vi "FPGA - Clear.vi"(8 "error in (no error)":errorcluster, 11 "Node Ptr":u64 format="%.0x") -> (0 "error out":errorcluster)   [LabVIEW 2011, in "Scan Engine Custom Device.lvlib"]
uses:
  Scan Engine Custom Device.lvlib
  Type Defs/FPGA Target.ctl
  Type Defs/Host - FPGAScanInterfaceMode.ctl
  Globals/Scan Engine GUIDs.vi
  <vilib>/NI Veristand/Custom Device API/Custom Device API.lvlib
  <vilib>/NI Veristand/Custom Device Tools/Custom Device Utility Library/Custom Device Utility Library.lvlib
panel:
  in  "Tag":string
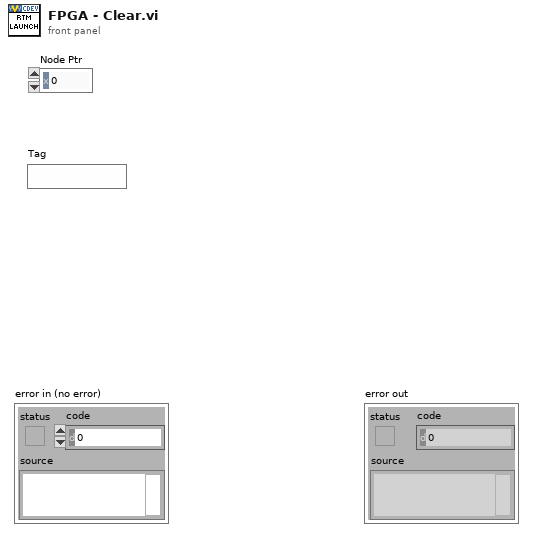
[diagram p1: front panel]
types:
  T1 = typedef "Scan Engine Custom Device.lvlib/Host - FPGAScanInterfaceMode.ctl" = enum16{"Use Current", "FPGA", "Scan Mode"}
  T2 = typedef "Scan Engine Custom Device.lvlib/FPGA Target.ctl" = enum16{"Local", "EtherCAT"}
  T3 = typedef "Custom Device API.lvlib/Custom Device Item Info.ctl" = cluster{"Name":string, "Is Channel":bool, "GUID":string}
  T4 = typedef "Custom Device API.lvlib/Custom Device Item Ref.ctl" = u64
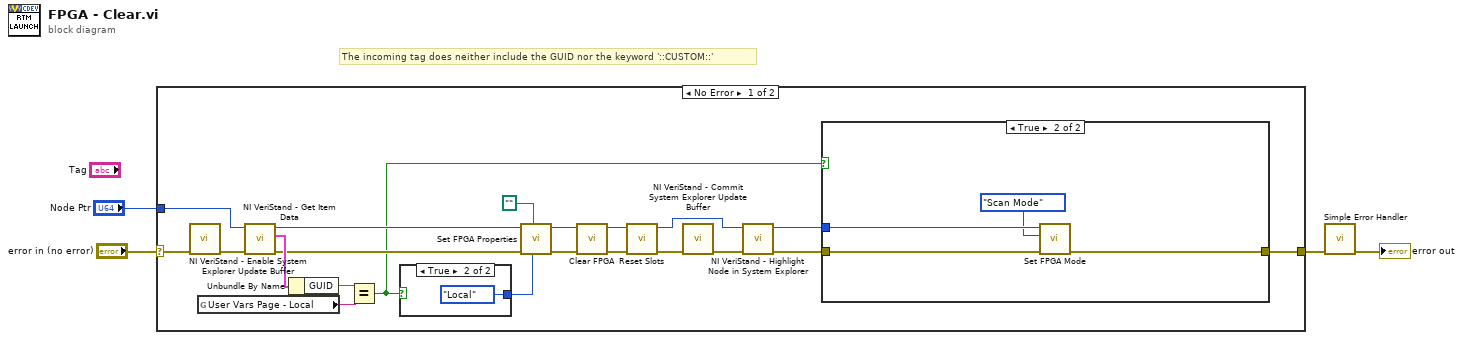
[diagram p0: block diagram]
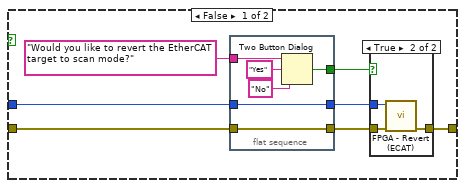
[diagram p2: hidden frame]
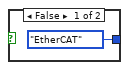
[diagram p4: hidden frame]
diagram:
  # "The incoming tag does neither include the GUID nor the keyword '::CUSTOM::'"
  n1 = case shown="No Error" "error in (no error)" {
    selector: "error in (no error)" -> [w19 w49]
    tunnel: "Node Ptr" -> [w13 _]
    tunnel: [w6 w49] -> w2
    frame No Error {
      n2 = call <vilib>:"NI VeriStand - Enable System Explorer Update Buffer.vi"("error in (no error)"=w19) -> ("error out"=w14:errorcluster)  [unwired: 10 in]
      n3 = global read "Scan Engine GUIDs.vi" "User Vars Page - Local"() -> (w10:string)
      n4 = call <vilib>:"NI VeriStand - Get Item Data.vi"("error in (no error)"=w14, "Item Ref in"=w13) -> ("error out"=w9:errorcluster, "Item Info"=w15:T3, "Item Ref out"=w12:T4)  [unwired: 6 in, 1 out]
      n5 = Unbundle By Name(w15) -> ("GUID"=w11:string)
      n6 = Equal?(x=w11, y=w10) -> (x = y?=w5:bool)
      n7 = case shown="True" w5 {
        tunnel: [FPGA_Target."EtherCAT" ("FPGA Target") FPGA_Target."Local" ("FPGA Target")] -> w23
        frame False {
        }
        frame True {
        }
      }
      n8 = call "Set FPGA Properties.vi"("FPGA Target"=w23, "Bitfile Path"=path "", "error in (no error)"=w9, "Item Ref in"=w12) -> ("error out"=w20:errorcluster, "Item Ref out"=w21:T4)  [unwired: 6 in]
      n9 = call "Clear FPGA.vi"("error in (no error)"=w20, "Item Ref in"=w21) -> ("error out"=w24:errorcluster, "Item Ref out"=w25:T4)  [unwired: 8 in]
      n10 = call "Reset Slots.vi"("error in (no error)"=w24, "Item Ref in"=w25) -> ("error out"=w18:errorcluster, "Item Ref out"=w16:T4)  [unwired: 8 in]
      n11 = call <vilib>:"NI VeriStand - Commit System Explorer Update Buffer.vi"("error in (no error)"=w18) -> ("error out"=w17:errorcluster)  [unwired: 10 in]
      n12 = call <vilib>:"NI VeriStand - Highlight Node in System Explorer.vi"("error in (no error)"=w17, "Item Ref in"=w16) -> ("error out"=w8:errorcluster, "Node Ptr dup"=w7:T4)  [unwired: 8 in]
      n13 = case shown="True" w5 {
        tunnel: w8 -> [w31 w46]
        tunnel: w7 -> [w30 w45]
        tunnel: [w27 w43] -> w6
        frame False {
          n14 = flat-sequence {
            tunnel: w31 -> [w40]
            tunnel: [w40] -> w28
            tunnel: "Would you like to revert the EtherCAT target to scan mode?" ("message") -> [w39]
            tunnel: [w38] -> w29
            tunnel: w30 -> [w38]
            tunnel: [w37] -> w26
            frame #0 {
              n15 = Two Button Dialog(message=w39, 1:"No" ("F button name (\"Cancel\")"), 2:"Yes" ("T button name (\"OK\")")) -> (T button?=w37:bool)
            }
          }
          n16 = case shown="True" w26 {
            tunnel: w28 -> [w33 w36]
            tunnel: w29 -> [_ w34]
            tunnel: [w33 w35] -> w27
            frame False {
            }
            frame True {
              n17 = call "FPGA - Revert (ECAT).vi"("error in (no error)"=w36, "Node Ptr"=w34) -> ("error out"=w35:errorcluster)  [unwired: 9 in]
            }
          }
        }
        frame True {
          n18 = call "Set FPGA Mode.vi"("error in (no error)"=w46, "FPGAScanInterfaceMode"=Host_-_FPGAScanInterfaceMode."Scan Mode", "Item Ref in"=w45) -> ("error out"=w43:errorcluster)  [unwired: 7 in, 1 out]
        }
      }
    }
    frame Error {
    }
  }
  n19 = call <vilib>:"Simple Error Handler.vi"("error in (no error)"=w2) -> ("error out"=→"error out":errorcluster)  [unwired: 4 in, 4 out]
